vi "Sum.vi"(11 "连接的字符串":string) -> (1 "字符串 3":string, 2 "string":string, 3 "无符号字节数组":u8[](array[numeric]))   [LabVIEW 2014]
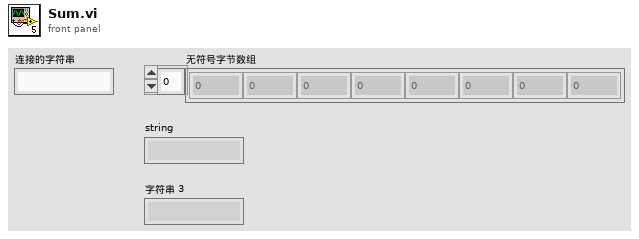
[diagram p1: front panel]
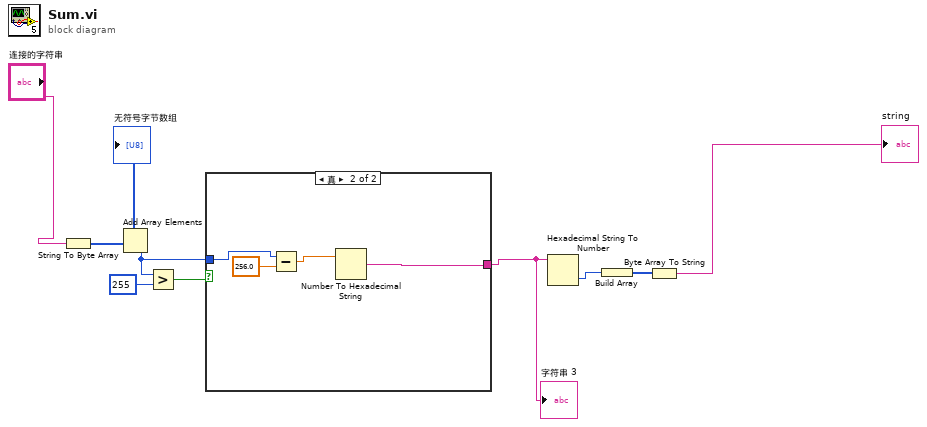
[diagram p0: block diagram]
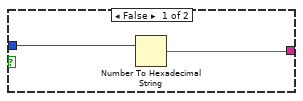
[diagram p2: hidden frame]
diagram:
  n1 = String To Byte Array(string="连接的字符串") -> (unsigned byte array=w7:u8[])
  "无符号字节数组" <- w7
  n2 = Add Array Elements(numeric array=w7) -> (sum=w4:u8)
  n3 = Greater?(x=w4, y=u8 255) -> (0:w5:bool)
  n4 = case shown="真" w5 {
    tunnel: w4 -> [w11 w14]
    tunnel: [w10 w12] -> w3
    frame False {
      n5 = Number To Hexadecimal String(2:w11) -> (0:w10:string)  [unwired: 1 in]
    }
    frame True {
      n6 = Subtract(x=w14, y=256.0) -> (x-y=w13:dbl)
      n7 = Number To Hexadecimal String(2:w13) -> (0:w12:string)  [unwired: 1 in]
    }
  }
  "字符串 3" <- w3
  n8 = Hexadecimal String To Number(string=w3) -> (number=w2:u32)  [unwired: 2 in, 1 out]
  n9 = Build Array(w2) -> (w1:u32[])
  n10 = Byte Array To String(unsigned byte array=w1) -> (string=→"string":string)
